vi "SVX9000NIModbus.vi"() -> ()   [LabVIEW 2011]
uses:
  <vilib>/NI Modbus.llb/MB Ethernet Master Query Write Single Register (poly).vi
  <vilib>/NI Modbus.llb/MB Ethernet Master Query Write Single Coil (poly).vi
panel:
  in  "Execute Profile":bool
  in  "Change Profile":u8(ring) items=["Select a Profile", "Closing Profile", "Opening Profile"]
  out "SVX Freq":dbl(graph)
  in  "Ramp":sgl=10.0 min=0 max=10 step=0.1 format="%.1f"
  in  "Ramp Shape":bool
  in  "Dec Time":sgl=30.0 min=0 max=6553.5 step=0.1 format="%.1f"
  in  "Decceleration Time":bool
  in  "Acc Time":sgl=30.0 min=0 max=6553.5 step=0.1 format="%.1f"
  in  "Acceleration Time":bool
  in  "left":bool
  in  "right":bool
  in  "Vel %":sgl=100.0 max=100 step=1
  in  "Velocity":bool
  in  "stop":bool
  in  "start":bool
  in  "Remote port":u16=502
  in  "Server address":string="192.168.1.3"
  in  "stop_app":bool
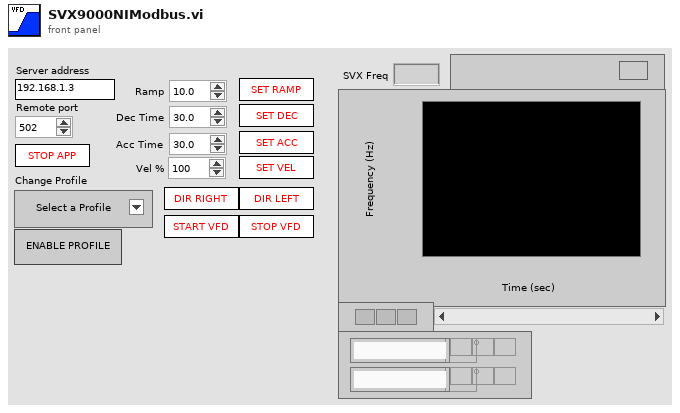
[diagram p1: front panel]
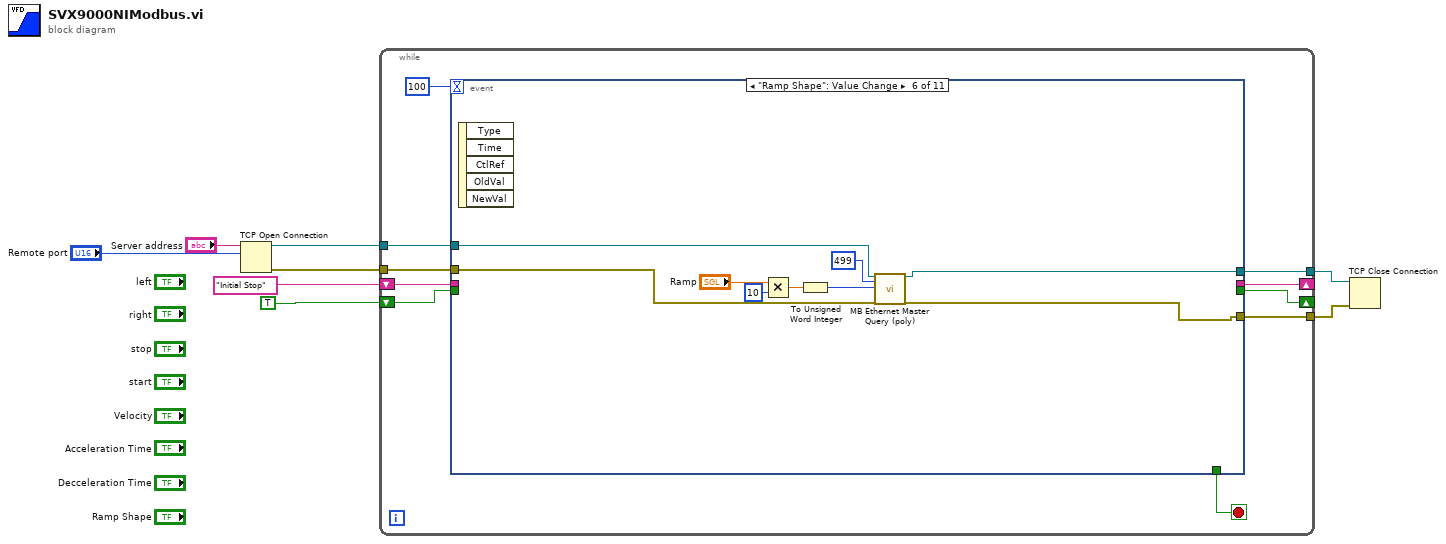
[diagram p0: block diagram]
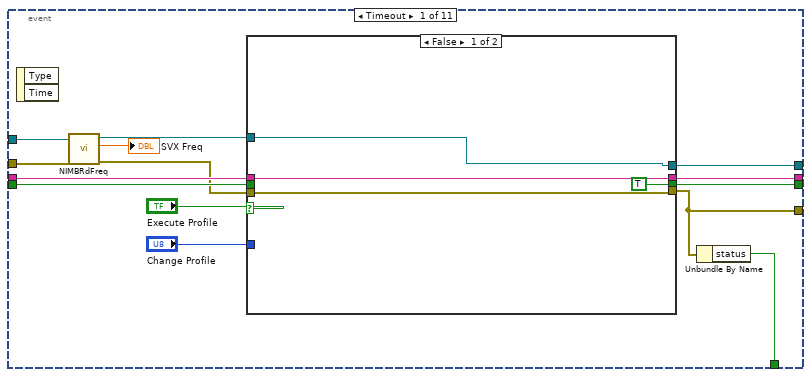
[diagram p2: hidden frame]
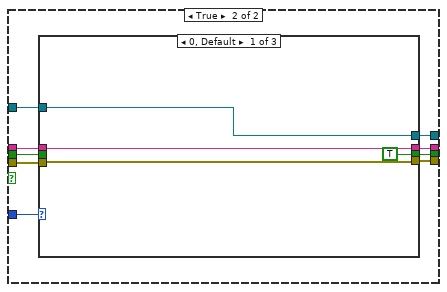
[diagram p3: hidden frame]
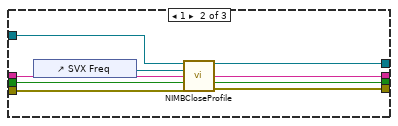
[diagram p4: hidden frame]
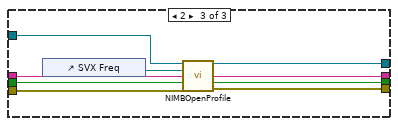
[diagram p5: hidden frame]
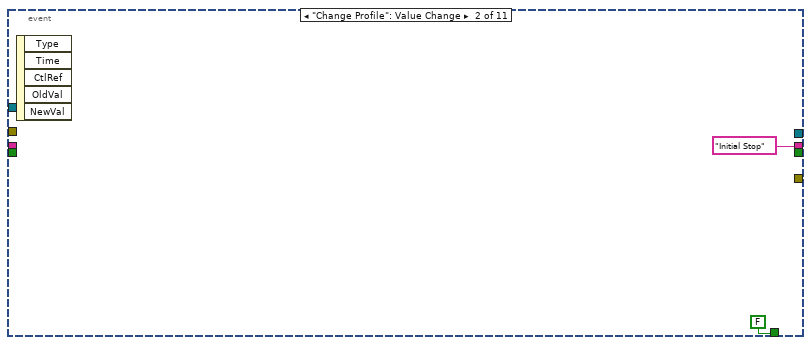
[diagram p6: hidden frame]
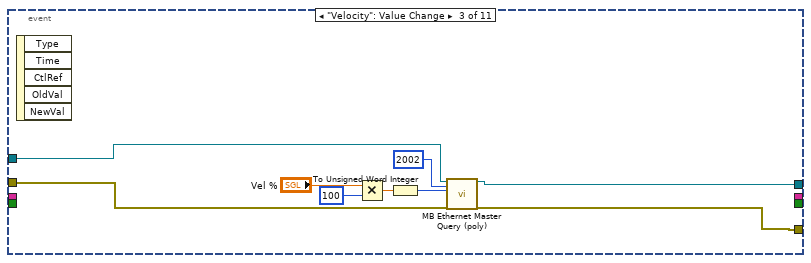
[diagram p7: hidden frame]
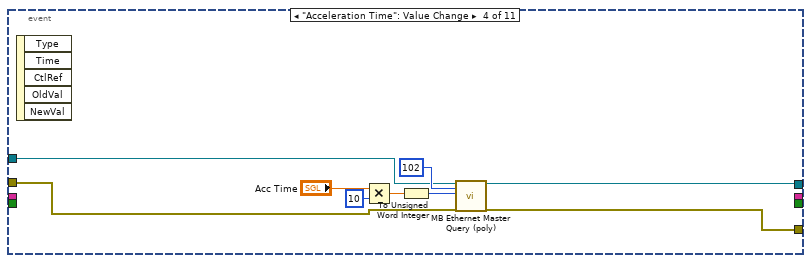
[diagram p8: hidden frame]
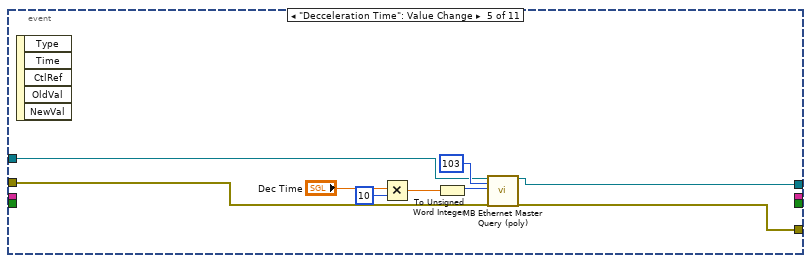
[diagram p9: hidden frame]
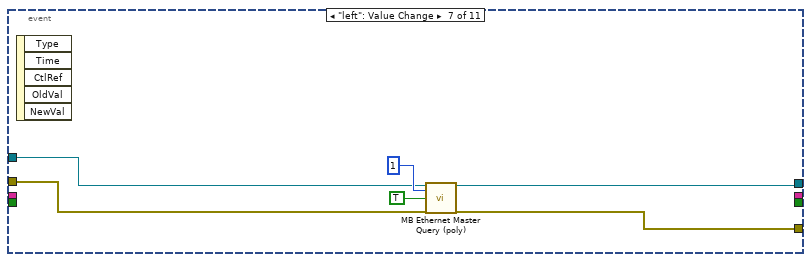
[diagram p10: hidden frame]
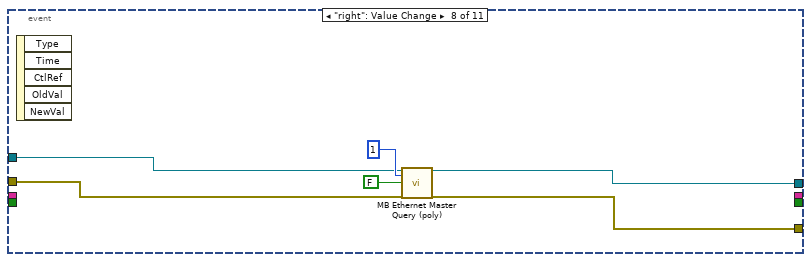
[diagram p11: hidden frame]
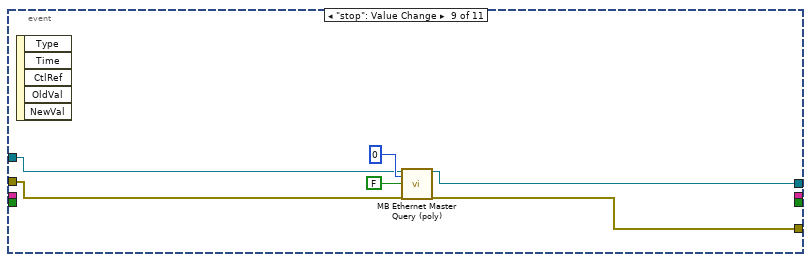
[diagram p12: hidden frame]
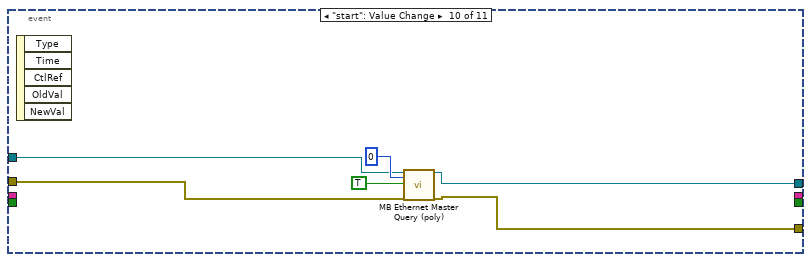
[diagram p13: hidden frame]
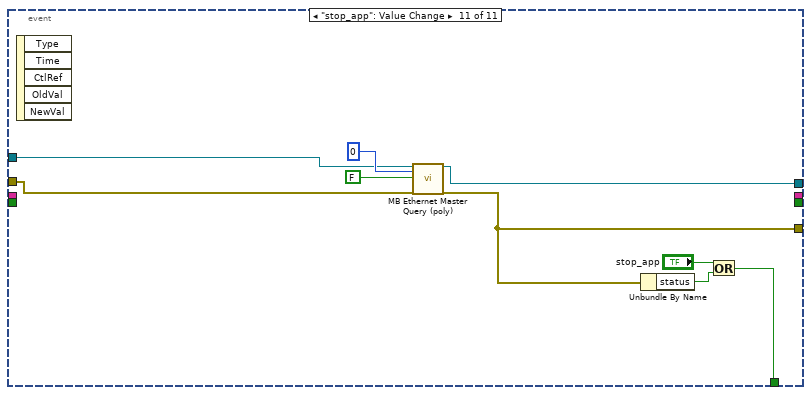
[diagram p14: hidden frame]
diagram:
  n1 = TCP Open Connection(address="Server address", remote port or service name="Remote port") -> (connection ID=w4:refnum<k5>, error out=w3:errorcluster)  [unwired: 3 in]
  n2 = while {
    shift-right: [w15] -> _
    shift-left: "Initial Stop" -> [w16]
    shift-right: [w13] -> _
    shift-left: TRUE -> [w14]
    tunnel: w4 -> [w12]
    tunnel: w3 -> [w11]
    tunnel: [w10] -> w2
    tunnel: [w9] -> w1
    stop <- w18 stop-if-true
    n3 = event shown="[5] \"Ramp Shape\": Value Change" {
      selector: _ -> [_ _ _ _ _ _ _ _ _ _ _]
      dyn-events: _ -> [_ _ _ _ _ _ _ _ _ _ _]
      timeout: 100 -> [_ _ _ _ _ _ _ _ _ _ _]
      tunnel: [w25 FALSE ("Error Flag") _ _ _ _ _ _ _ _ w136] -> w18
      tunnel: w16 -> [w32 _ _ _ _ _ _ _ _ _ _]
      tunnel: [w31 "Initial Stop" _ _ _ _ _ _ _ _ _] -> w15
      tunnel: [w28 _ _ _ _ _ _ _ _ _ _] -> w13
      tunnel: w14 -> [w27 _ _ _ _ _ _ _ _ _ _]
      tunnel: w12 -> [w23 _ w73 w82 w91 w100 w109 w115 w121 w127 w133]
      tunnel: w11 -> [w22 _ w72 w81 w90 w99 w108 w114 w120 w126 w132]
      tunnel: [w20 _ w71 w80 w89 w98 w107 w113 w119 w125 w131] -> w10
      tunnel: [w19 _ w70 w79 w88 w97 w106 w112 w118 w124 w130] -> w9
      event Timeout {
        n4 = event-data() -> ()  [unwired: 1 in, 2 out]
        n5 = call "NIMBRdFreq.vi"("error in (no error)"=w22, "TCP Network Connection in"=w23) -> ("error out"=w21:errorcluster, "Output Frequency"=→"SVX Freq":dbl, "TCP Network Connection out"=w24:refnum<k5>)  [unwired: 2 in, 1 out]
        n6 = case shown="False" "Execute Profile" {
          tunnel: w32 -> [w36 w45]
          tunnel: [w36 w44] -> w31
          tunnel: "Change Profile" -> [_ w43]
          tunnel: w24 -> [w33 w42]
          tunnel: [TRUE w41] -> w28
          tunnel: w27 -> [_ w40]
          tunnel: [w34 w39] -> w19
          tunnel: w21 -> [w34 w38]
          tunnel: [w33 w37] -> w20
          frame False {
          }
          frame True {
            n7 = case shown="0, Default" w43 {
              tunnel: w45 -> [w49 w56 w65]
              tunnel: [w49 w54 w60] -> w44
              tunnel: w42 -> [w46 w57 w66]
              tunnel: [TRUE w53 w61] -> w41
              tunnel: w40 -> [_ w55 w64]
              tunnel: [w47 w52 w62] -> w39
              tunnel: w38 -> [w47 w51 w63]
              tunnel: [w46 w50 w59] -> w37
              frame 0, Default {
              }
              frame 1 {
                n8 = control-ref of="SVX Freq"() -> (w58:refnum<vi>)
                n9 = call "NIMBCloseProfile.vi"("connection ID"=w57, "WaveformChart in"=w58, "String in"=w56, "Boolean in"=w55, "error in"=w51) -> ("TCP Connection Refnum (dup)"=w50:refnum<k5>, "String out"=w54:string, "Boolean out"=w53:bool, "error out"=w52:errorcluster)  [unwired: 7 in]
              }
              frame 2 {
                n10 = control-ref of="SVX Freq"() -> (w67:refnum<vi>)
                n11 = call "NIMBOpenProfile.vi"("connection ID"=w66, "WaveformChart in"=w67, "String in"=w65, "Boolean in"=w64, "error in"=w63) -> ("connection ID out"=w59:refnum<k5>, "String out"=w60:string, "Boolean out"=w61:bool, "error out"=w62:errorcluster)  [unwired: 7 in]
              }
            }
          }
        }
        n12 = Unbundle By Name(w19) -> ("status"=w25:bool)
      }
      event "Change Profile": Value Change {
        n13 = event-data() -> ()  [unwired: 1 in, 5 out]
      }
      event "Velocity": Value Change {
        n14 = event-data() -> ()  [unwired: 1 in, 5 out]
        n15 = Multiply(x="Vel %", y=u8 100) -> (x*y=w75:sgl)
        n16 = To Unsigned Word Integer(number=w75) -> (unsigned 16bit integer=w74:u16)
        n17 = call-poly <vilib>:"MB Ethernet Master Query (poly).vi"("TCP Connection Refnum in"=w73, "Address"=u16 2002 ("MB Reg No"), "Register"=w74, "error in"=w72) -> ("TCP Connection Refnum (dup)"=w71:refnum<k5>, "error out"=w70:errorcluster)  [unwired: 13 in, 1 out]
      }
      event "Acceleration Time": Value Change {
        n18 = event-data() -> ()  [unwired: 1 in, 5 out]
        n19 = Multiply(x="Acc Time", y=u8 10) -> (x*y=w85:sgl)
        n20 = To Unsigned Word Integer(number=w85) -> (unsigned 16bit integer=w86:u16)
        n21 = call-poly <vilib>:"MB Ethernet Master Query (poly).vi"("TCP Connection Refnum in"=w82, "Address"=u16 102 ("Word address"), "Register"=w86, "error in"=w81) -> ("TCP Connection Refnum (dup)"=w80:refnum<k5>, "error out"=w79:errorcluster)  [unwired: 13 in, 1 out]
      }
      event "Decceleration Time": Value Change {
        n22 = event-data() -> ()  [unwired: 1 in, 5 out]
        n23 = Multiply(x="Dec Time", y=u8 10) -> (x*y=w92:sgl)
        n24 = To Unsigned Word Integer(number=w92) -> (unsigned 16bit integer=w96:u16)
        n25 = call-poly <vilib>:"MB Ethernet Master Query (poly).vi"("TCP Connection Refnum in"=w91, "Address"=u16 103 ("Word address"), "Register"=w96, "error in"=w90) -> ("TCP Connection Refnum (dup)"=w89:refnum<k5>, "error out"=w88:errorcluster)  [unwired: 13 in, 1 out]
      }
      event "Ramp Shape": Value Change {
        n26 = event-data() -> ()  [unwired: 1 in, 5 out]
        n27 = Multiply(x="Ramp", y=u8 10) -> (x*y=w104:sgl)
        n28 = To Unsigned Word Integer(number=w104) -> (unsigned 16bit integer=w102:u16)
        n29 = call-poly <vilib>:"MB Ethernet Master Query (poly).vi"("TCP Connection Refnum in"=w100, "Address"=u16 499 ("Word address"), "Register"=w102, "error in"=w99) -> ("TCP Connection Refnum (dup)"=w98:refnum<k5>, "error out"=w97:errorcluster)  [unwired: 13 in, 1 out]
      }
      event "left": Value Change {
        n30 = event-data() -> ()  [unwired: 1 in, 5 out]
        n31 = call-poly <vilib>:"MB Ethernet Master Query (poly).vi"("TCP Connection Refnum in"=w109, "Address"=u8 1 ("MB Reg No"), "Coil"=TRUE ("Bit"), "error in"=w108) -> ("TCP Connection Refnum (dup)"=w107:refnum<k5>, "error out"=w106:errorcluster)  [unwired: 13 in, 1 out]
      }
      event "right": Value Change {
        n32 = event-data() -> ()  [unwired: 1 in, 5 out]
        n33 = call-poly <vilib>:"MB Ethernet Master Query (poly).vi"("TCP Connection Refnum in"=w115, "Address"=u8 1 ("MB Reg No"), "Coil"=FALSE ("Bit"), "error in"=w114) -> ("TCP Connection Refnum (dup)"=w113:refnum<k5>, "error out"=w112:errorcluster)  [unwired: 13 in, 1 out]
      }
      event "stop": Value Change {
        n34 = event-data() -> ()  [unwired: 1 in, 5 out]
        n35 = call-poly <vilib>:"MB Ethernet Master Query (poly).vi"("TCP Connection Refnum in"=w121, "Address"=u8 0 ("MB Reg No"), "Coil"=FALSE ("Bit"), "error in"=w120) -> ("TCP Connection Refnum (dup)"=w119:refnum<k5>, "error out"=w118:errorcluster)  [unwired: 13 in, 1 out]
      }
      event "start": Value Change {
        n36 = event-data() -> ()  [unwired: 1 in, 5 out]
        n37 = call-poly <vilib>:"MB Ethernet Master Query (poly).vi"("TCP Connection Refnum in"=w127, "Address"=u8 0 ("MB Reg No"), "Coil"=TRUE ("Bit"), "error in"=w126) -> ("TCP Connection Refnum (dup)"=w125:refnum<k5>, "error out"=w124:errorcluster)  [unwired: 13 in, 1 out]
      }
      event "stop_app": Value Change {
        n38 = event-data() -> ()  [unwired: 1 in, 5 out]
        n39 = call-poly <vilib>:"MB Ethernet Master Query (poly).vi"("TCP Connection Refnum in"=w133, "Address"=u16 0 ("MB Reg No"), "Coil"=FALSE ("Bit"), "error in"=w132) -> ("TCP Connection Refnum (dup)"=w131:refnum<k5>, "error out"=w130:errorcluster)  [unwired: 13 in, 1 out]
        n40 = Unbundle By Name(w130) -> ("status"=w134:bool)
        n41 = Or(x="stop_app", y=w134) -> (x .or. y?=w136:bool)
      }
    }
  }
  n42 = TCP Close Connection(connection ID=w2, error in (no error)=w1) -> ()  [unwired: 1 in, 2 out]
